vi "check_frequency_sweepII_parameters.vi"(8 "error in (no error)":errorcluster, 10 "Frequency Sweep II Parameters 2":T1={"f (Hz)"=0.0, "Number of steps"=2, "Total time (s)"=0.0, "fc_start (Hz)"=2000.0, "Modulation Depth (0.0 %)"=0.0, "Channel (1:Channel 1)"=2, "fc_end (Hz)"=2000.0, "amp (V)"=1.0, "DC Offset (V)"=0.0} {"DC Offset (V)" min=-20.0 max=20.0 format="%#_13g"; "amp (V)" min=0.0 max=20.0 format="%#_13g"; "fc_end (Hz)" min=0.0 format="%#_13g"; "Channel (1:Channel 1)" items=["Channel 1"=1, "Channel 2"=2]; "Modulation Depth (0.0 %)" min=0.0 max=120.0 format="%.1f"; "fc_start (Hz)" min=0.0 format="%#_13g"; "Total time (s)" min=0.0; "Number of steps" min=2; "f (Hz)" min=0.0}) -> (0 "error out":errorcluster, 1 "Array":dbl[](array[numeric]), 2 "Entered Values OK":bool)   [LabVIEW 2024, in "Sweep.lvlib"]
uses:
  Sweep.lvlib
  Type Definitions/Frequency_sweep_II Parameters.ctl
panel:
  out "fc_end (Hz) 2":dbl
  out "fc_start (Hz)":dbl
  out "Number of frequencies":i32
  out "Total time T (s)":dbl
  out "Channel (1:Channel 1)":i32
  out "Modulation Depth (0.0 %)":dbl
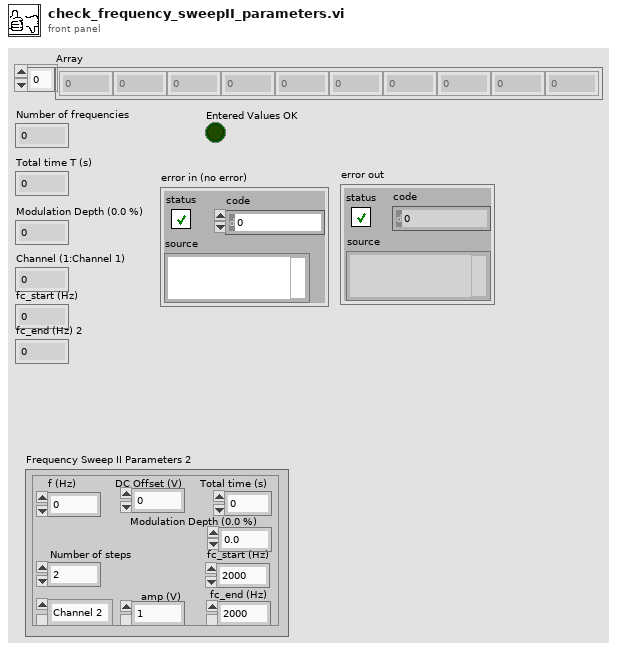
[diagram p1: front panel]
types:
  T1 = typedef "Frequency_sweep_II Parameters.ctl" = cluster{"f (Hz)":dbl, "Number of steps":i32, "Total time (s)":dbl, "fc_start (Hz)":dbl, "Modulation Depth (0.0 %)":dbl, "Channel (1:Channel 1)":i32, "fc_end (Hz)":dbl, "amp (V)":dbl, "DC Offset (V)":dbl}
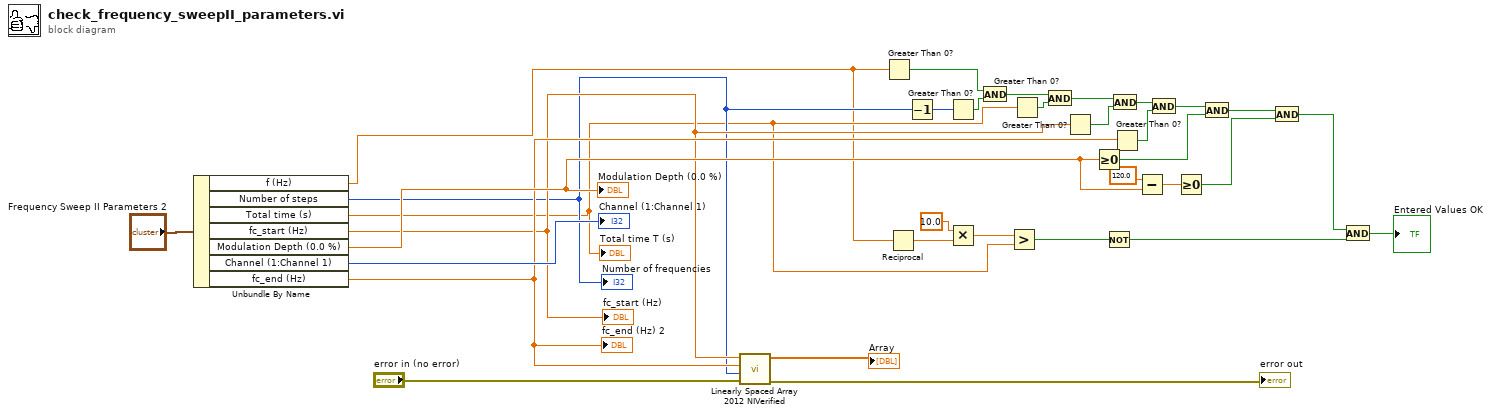
[diagram p0: block diagram]
diagram:
  n1 = Unbundle By Name("Frequency Sweep II Parameters 2") -> ("f (Hz)"=w1:dbl, "Number of steps"=w3:i32, "Total time (s)"=w2:dbl, "fc_start (Hz)"=w4:dbl, "Modulation Depth (0.0 %)"=w7:dbl, "Channel (1:Channel 1)"=→"Channel (1:Channel 1)":i32, "fc_end (Hz)"=w5:dbl)
  "Modulation Depth (0.0 %)" <- w7
  "Total time T (s)" <- w2
  "Number of frequencies" <- w3
  "fc_start (Hz)" <- w4
  "fc_end (Hz) 2" <- w5
  n2 = call "Linearly Spaced Array 2012 NIVerified.vi"("error in (no error)"="error in (no error)", "Number of Samples"=w3, "End"=w5, "Start"=w4) -> ("error out"=→"error out":errorcluster, "Array"=→"Array":dbl[])  [unwired: 6 in]
  n3 = Greater Than 0?(x=w1) -> (x > 0?=w23:bool)
  n4 = Reciprocal(x=w1) -> (1/x=w10:dbl)
  n5 = Decrement(x=w3) -> (x-1=w19:i32)
  n6 = Greater Than 0?(x=w19) -> (x > 0?=w24:bool)
  n7 = Multiply(x=10.0, y=w10) -> (x*y=w31:dbl)
  n8 = And(x=w23, y=w24) -> (x .and. y?=w25:bool)
  n9 = Greater?(x=w31, y=w2) -> (0:w32:bool)
  n10 = Greater Than 0?(x=w2) -> (x > 0?=w26:bool)
  n11 = And(x=w25, y=w26) -> (x .and. y?=w27:bool)
  n12 = Greater Than 0?(x=w4) -> (x > 0?=w28:bool)
  n13 = Greater Or Equal To 0?(x=w7) -> (x >= 0?=w18:bool)
  n14 = Not(x=w32) -> (.not. x?=w33:bool)
  n15 = And(x=w27, y=w28) -> (x .and. y?=w30:bool)
  n16 = Greater Than 0?(x=w5) -> (x > 0?=w11:bool)
  n17 = Subtract(x=120.0, y=w7) -> (x-y=w15:dbl)
  n18 = And(x=w30, y=w11) -> (x .and. y?=w12:bool)
  n19 = Greater Or Equal To 0?(x=w15) -> (x >= 0?=w14:bool)
  n20 = And(x=w12, y=w18) -> (x .and. y?=w16:bool)
  n21 = And(x=w16, y=w14) -> (x .and. y?=w17:bool)
  n22 = And(x=w17, y=w33) -> (x .and. y?=→"Entered Values OK":bool)
